vi "SetAuthority.vi"(6 "Sequence Number (16 bits)":u16=1, 7 "QueryType":u8=2) -> (3 "Encoded JAUS Message":string)   [LabVIEW 2009]
uses:
  Support Files/Address.ctl
panel:
  in  "Destination":T1={"Subsystem Id"=90, "Node Id"=1, "Component Id"=1}
  in  "Source":T1={"Subsystem Id"=3, "Node Id"=1, "Component Id"=1}
  in  "Command Code":string="\u0000\u0001"
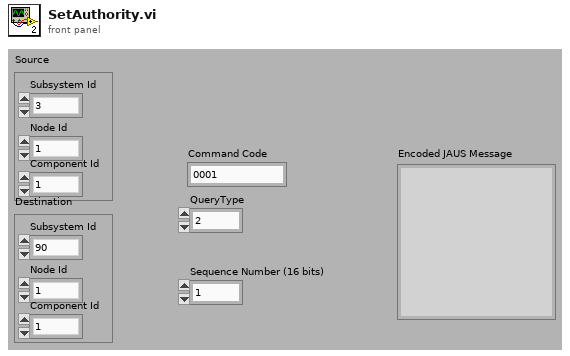
[diagram p1: front panel]
types:
  T1 = typedef "Address.ctl" = cluster{"Subsystem Id":u16, "Node Id":u8, "Component Id":u8}
  T2 = cluster{"unsigned byte array[0]":u8, "unsigned byte array[1]":u8}
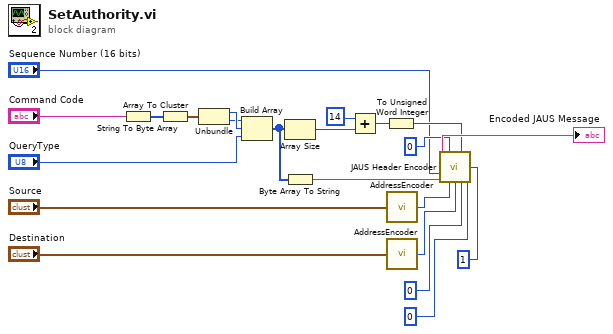
[diagram p0: block diagram]
diagram:
  n1 = String To Byte Array(string="Command Code") -> (unsigned byte array=w8:u8[])
  n2 = Array To Cluster(array=w8) -> (cluster=w7:T2)
  n3 = Unbundle(w7) -> ("unsigned byte array[0]"=w6:u8, "unsigned byte array[1]"=w5:u8)
  n4 = Build Array(w5, w6, "QueryType") -> (w12:u8[])
  n5 = Array Size(array=w12) -> (size(s)=w10:i32)
  n6 = Byte Array To String(unsigned byte array=w12) -> (string=w14:string)
  n7 = Add(x=14, y=w10) -> (x+y=w9:i32)
  n8 = To Unsigned Word Integer(number=w9) -> (unsigned 16bit integer=w2:u16)
  n9 = call "AddressEncoder.vi"("Address Cluster"="Source") -> ("Address"=w21:u32)
  n10 = call "AddressEncoder.vi"("Address Cluster"="Destination") -> ("Address"=w20:u32)
  n11 = call "JAUS Header Encoder.vi"("Message Type (0-5)"=u8 0, "Data Size (8-23)"=w2, "Priority(40-41)"=u8 1, "Sequence Number (16 bits)"="Sequence Number (16 bits)", "Payload"=w14, "Source ID (80-95)"=w21, "Destination ID (48-79)"=w20, "Data Flags (46-47)"=u8 0, "Ack/Nak (44-45)"=u8 0) -> ("Encoded JAUS Message"=→"Encoded JAUS Message":string)  [unwired: 6 in]
